vi "StartAutoMode.vi"(8 "error in (no error)":errorcluster, 11 "MainData":T1) -> (0 "error out":errorcluster, 3 "MainData out":T1)   [LabVIEW 2019, in "MainController.lvlib"]
uses:
  MainController.lvlib
  Cluster - MainData.ctl
  All Message Queues.ctl
  Cluster - MainControllerMessage.ctl
  Enum - MainState.ctl
  AutoMode/Cluster - AutoModeMessage.ctl
  AutoMode/Enum - AutoModeState.ctl
  ManualMode/Cluster - ManualModeMessageCluster.ctl
  ManualMode/Enum - ManualModeMessage.ctl
  Settings/CTL_MessageCluster.ctl
  Settings/CTL_SettingsMessage.ctl
  EventLogger/Cluster - MessageCluster.ctl
  EventLogger/Enum - Message.ctl
  Cluster - HardwareConfiguration.ctl
  Cluster - LoggingConfiguration.ctl
  Cluster - TestSettings.ctl
  UI State.ctl
  UI Data.ctl
  AutoMode/AutoMode.lvlib
  EventLogger/EventLogger.lvlib
  ManualMode/ManualMode.lvlib
  Settings/Settings.lvlib
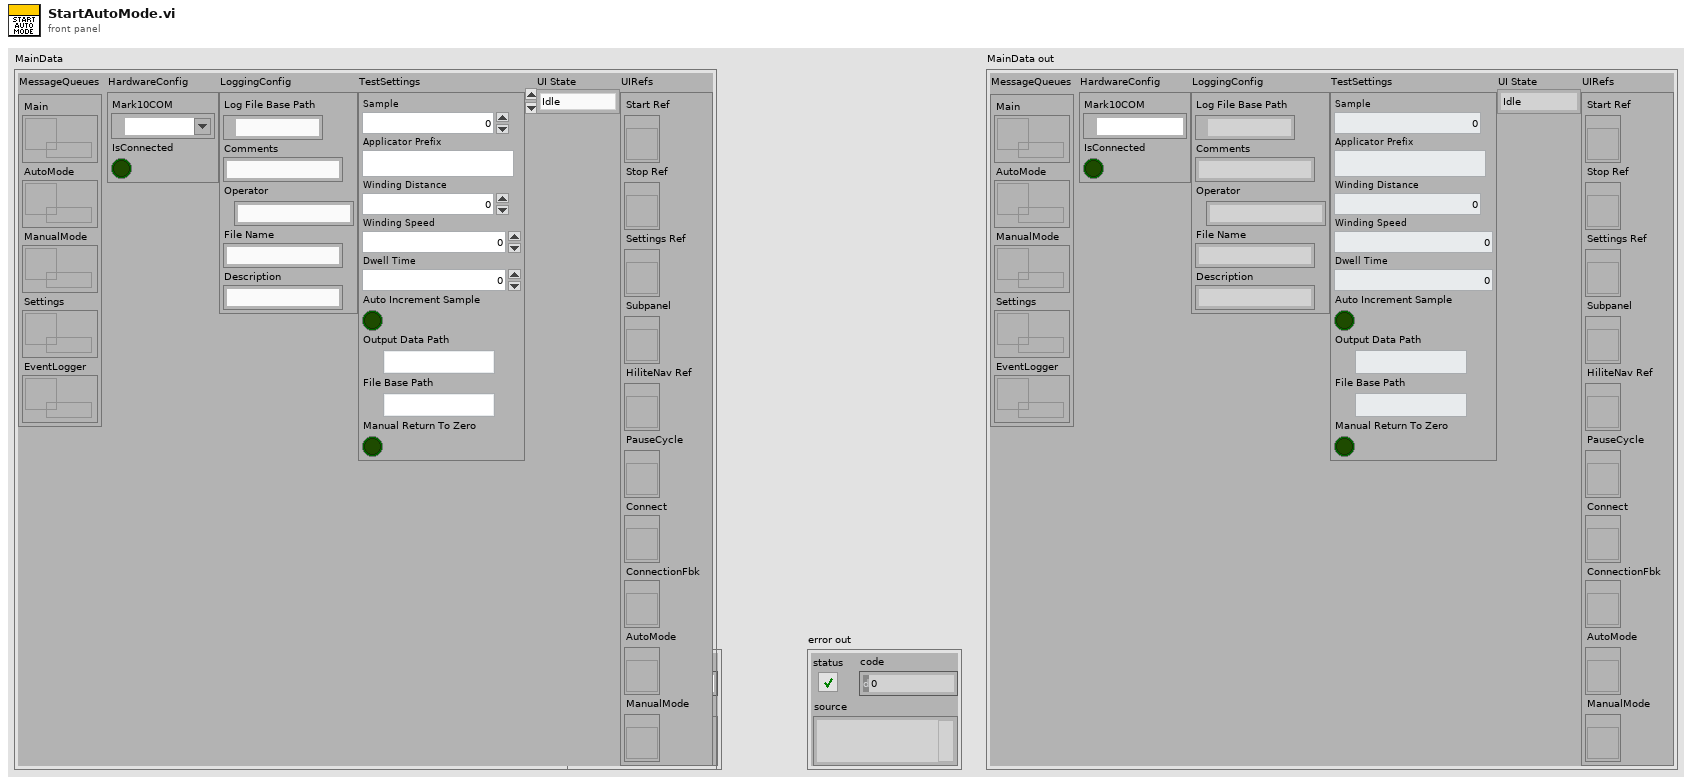
[diagram p1: front panel]
types:
  T1 = typedef "MainController.lvlib/Cluster - MainData.ctl" = cluster{"MessageQueues":T2, "HardwareConfig":T3, "LoggingConfig":T4, "TestSettings":T5, "UI State":T6, "UIRefs":T7}
  T2 = typedef "MainController.lvlib/All Message Queues.ctl" = cluster{"Main":refnum<queue>, "AutoMode":refnum<queue>, "ManualMode":refnum<queue>, "Settings":refnum<queue>, "EventLogger":refnum<queue>}
  T3 = typedef "MainController.lvlib/Cluster - HardwareConfiguration.ctl" = cluster{"Mark10COM":refnum<visa-resource-name>, "IsConnected":bool}
  T4 = typedef "MainController.lvlib/Cluster - LoggingConfiguration.ctl" = cluster{"Log File Base Path":path, "Comments ":string, "Operator":string, "File Name":string, "Description":string}
  T5 = typedef "MainController.lvlib/Cluster - TestSettings.ctl" = cluster{"Sample":u32, "Applicator Prefix":string, "Winding Distance":dbl, "Winding Speed":dbl, "Dwell Time":dbl, "Auto Increment Sample":bool, "Output Data Path":path, "File Base Path":path, "Manual Return To Zero":bool}
  T6 = typedef "MainController.lvlib/UI State.ctl" = enum16{"Idle", "AutoIdle", "AutoRunning", "ManualMode", "Settings"}
  T7 = typedef "MainController.lvlib/UI Data.ctl" = cluster{"Start Ref":refnum<vi>, "Stop Ref":refnum<vi>, "Settings Ref":refnum<vi>, "Subpanel":refnum<vi>, "HiliteNav Ref":refnum<vi>, "PauseCycle":refnum<vi>, "Connect":refnum<vi>, "ConnectionFbk":refnum<vi>, "AutoMode":refnum<vi>, "ManualMode":refnum<vi>}
  T8 = typedef "MainController.lvlib/Enum - MainState.ctl" = enum16{"Initialize", "InitUIRefs", "LaunchSettings", "LaunchAutoMode", "LaunchManualMode", "LaunchTestReport", "ConnectHardware", "DisconnectHardware", "HiliteNavItems", "StartAutoMode", "PauseAutoMode", "StopAutoMode", "ShowFlyout", "HideFlyout", "BroadcastSettings", "PickupTestSettings", "BroadcastHW", "AutoTestDone", "DAQStatus", "UpdateCommandBar", "Error", "RecieveError", "Exit"}
  T9 = typedef "AutoMode.lvlib/Enum - AutoModeState.ctl" = enum16{"Initialize", "Idle", "UpdateConfig", "UpdateHWConfig", "BroadcastSettings", "Start", "CheckValidReportPath", "Winding", "WaitForWinding", "Unwind", "WaitForUnwind", "Stop", "Abort", "WriteDataToFile", "EventTriggered", "GenerateFilePath", "ZeroPosition", "GotoZero", "Error", "Exit"}
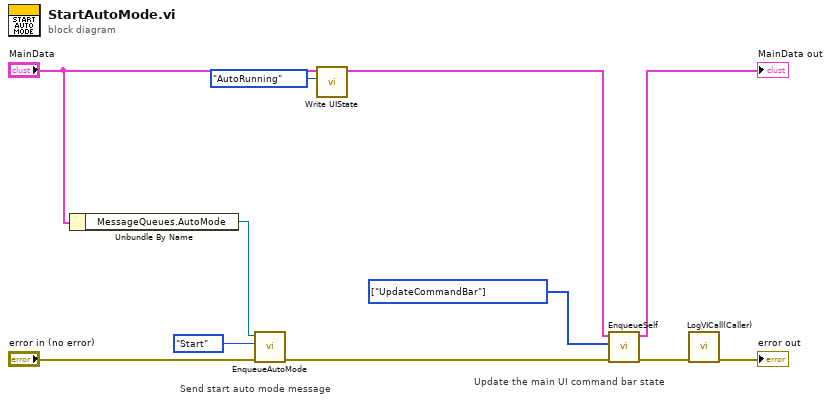
[diagram p0: block diagram]
diagram:
  w4 = T8[] [enum."UpdateCommandBar"] items=["Initialize", "InitUIRefs", "LaunchSettings", "LaunchAutoMode", "LaunchManualMode", "LaunchTestReport", "ConnectHardware", "DisconnectHardware", "HiliteNavItems", "StartAutoMode", "PauseAutoMode", "StopAutoMode", "ShowFlyout", "HideFlyout", "BroadcastSettings", "PickupTestSettings", "BroadcastHW", "AutoTestDone", "DAQStatus", "UpdateCommandBar", "Error", "RecieveError", "Exit"] ("Messages")
  # "Update the main UI command bar state"
  # "Send start auto mode message"
  n1 = Unbundle By Name("MainData") -> ("MessageQueues.AutoMode"=w8:refnum<queue>)
  n2 = call "EnqueueAutoMode.vi"("error in (no error)"="error in (no error)", "AutoState"=Enum_-_AutoModeState."Start" ("CycleTestState"), "Queue in"=w8) -> ("error out"=w10:errorcluster)  [unwired: 7 in, 1 out]
  n3 = call "Write UIState.vi"("UI State"=UI_State."AutoRunning", "MainData"="MainData") -> ("MainData out"=w3:T1)  [unwired: 9 in]
  n4 = call "EnqueueSelf.vi"("Error In"=w10, "Messages"=w4, "MainData"=w3) -> ("Error Out"=w7:errorcluster, "MainData out"=→"MainData out":T1)  [unwired: 7 in]
  n5 = call "LogVICall(Caller).vi"("Error In"=w7) -> ("Error Out"=→"error out":errorcluster)  [unwired: 10 in]
